vi "Do.vi"(8 "error in":errorcluster, 10 "Actor in":refnum<class "Actor.lvclass">, 11 "Start PAS Wvfm Save MSG":refnum<class "Start CRD RD File MSG.lvclass">) -> (0 "error out":errorcluster, 2 "Actor out":refnum<class "Actor.lvclass">)   [LabVIEW 2014, in "Controller.lvlib" / "Start CRD RD File MSG.lvclass"]
doc: "(<B>Filename</B>: Actor Framework.lvlib:Message.lvclass:Do.vi)\n\nDefines what a message does when it is received by an actor. Generally, a message instructs an actor to invoke one of its methods. By default, this method does nothing. A child class must override it to define behavior. Create a child class by using the Actor Framework Message Maker dialog box."
uses:
  Start CRD RD File MSG.lvclass
  <vilib>/ActorFramework/Actor/Actor.lvclass
  Controller.lvclass
  Controller.lvclass/Controller.ctl
  File Actor/File Actor.lvclass
  Exe CRD RD Write/Exe Write CRD RDs.lvclass
  Instr Exe Write to File/Instr Exe Write to File.lvclass/Instr Exe Write to File.ctl
  SuperActor/SuperActor.lvclass/SuperActor.ctl
  File Actor/File Actor.lvclass/File Actor.ctl
  SuperActor/Write ID.vi
  File Actor/Write Cfg Header.vi
  File Actor/Write Exe Write.vi
  File Actor/Write Wait on Registration_.vi
  Instr Exe Write to File/Write MAP DVR.vi
  Instr Exe Write to File/Write DataObj.vi
  Accessors/Read Data Map.vi
  File Actor/Write Registration Complete.vi
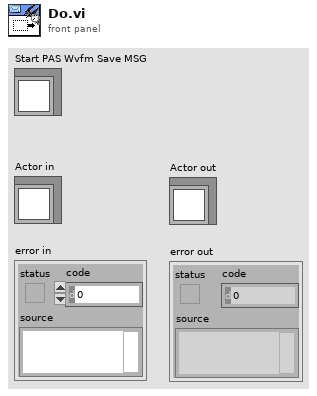
[diagram p1: front panel]
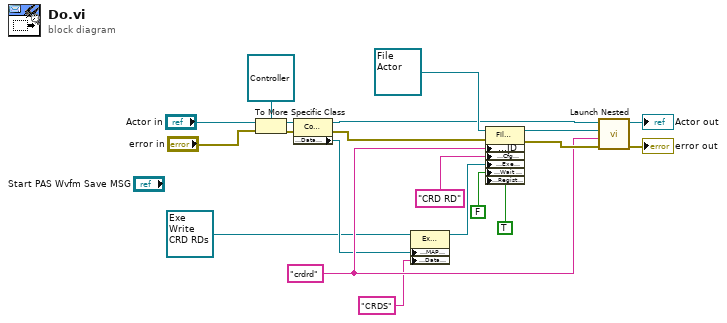
[diagram p0: block diagram]
diagram:
  w12 = "crdrd" ("ID")
  n1 = To More Specific Class(target class=refnum<class "Controller.lvclass"> refnum ("Controller:Controller"), reference="Actor in", error in="error in") -> (specific class reference=w10:refnum<class "Controller.lvclass">, error out=w9:errorcluster)
  n2 = property class="Controller"(reference=w10, error in=w9) -> (reference out=w8:refnum<class "Controller.lvclass">, error out=w7:errorcluster, "Accessors:Data Map"=w6:refnum<data-value>)
  n3 = property class="Exe Write PAS Wvfms"(reference=refnum<class "Exe Write CRD RDs.lvclass"> refnum ("Controller:Exe Write PAS Wvfms"), "Accessors:MAP DVR"=w6, "Accessors:DataObj"="CRDS" ("DataObj")) -> (reference out=w5:refnum<class "Exe Write CRD RDs.lvclass">)  [unwired: 1 in, 1 out]
  n4 = property class="File Actor"(reference=refnum<class "File Actor.lvclass"> refnum ("File Library.lvlib:File Actor"), error in=w7, "Accessors:ID"=w12, "Accessors:Cfg Header"="CRD RD" ("Cfg Header"), "Accessors:Exe Write"=w5, "Accessors:Wait on Registration_"=FALSE ("Wait on Registration_"), "Accessors:Registration Complete"=TRUE ("Registration Complete")) -> (reference out=w16:refnum<class "File Actor.lvclass">, error out=w15:errorcluster)
  n5 = call "Launch Nested.vi"("Error In"=w15, "ID"=w12, "Nested Actor"=w16, "Controller in"=w8) -> ("Error Out"=→"error out":errorcluster, "Controller out"=→"Actor out":refnum<class "Controller.lvclass">)  [unwired: 5 in, 1 out]
